vi "Main.vi"() -> ()   [LabVIEW 2014, in "CSV Analyzer.lvlib"]
uses:
  CSV Analyzer.lvlib
  <vilib>/SLL/SLL Table/SLL Table.lvclass
  <vilib>/Utility/error.llb/DialogType.ctl
  <vilib>/SLL/SLL Queued State Machine/Queue Driver/Create Queue.vi
  <vilib>/SLL/SLL Queued State Machine/Queue Driver/Enqueue an Item to Queue.vi
  <vilib>/SLL/SLL Queued State Machine/Queue Driver/Dequeue Queue.vi
  <vilib>/Utility/file.llb/Read From Spreadsheet File (string).vi
  <vilib>/SLL/SLL Queued State Machine/Queue Driver/Enqueue N Items.vi
  <vilib>/SLL/SLL Queued State Machine/Queue Driver/Flush Queue.vi
  <vilib>/SLL/SLL Queued State Machine/Queue Driver/Release Queue.vi
  <vilib>/SLL/SLL Queued State Machine/SLL QSM.lvlib
  <vilib>/SLL/SLL Spreadsheet/SLL Spreadsheet.lvlib
panel:
  in  "Delimiter":string(combo)=","
  in  "Use LabVIEW File Read?":bool
  in  "CSV File Path":path
  out "Total Columns":i32
  out "Total Rows":i32
  in  "Headers to List[]":string[](array[combo])
  in  "Filters":T1(array[cluster])
  out "Status":string
  in  "Count Rows":bool
  in  "Mini Table":bool
  out "Displayed Column Count":i32
  out "Displayed Row Count":i32
  in  "2D Data Out[][]":i32(listbox)
  # "CSV Analyzer"
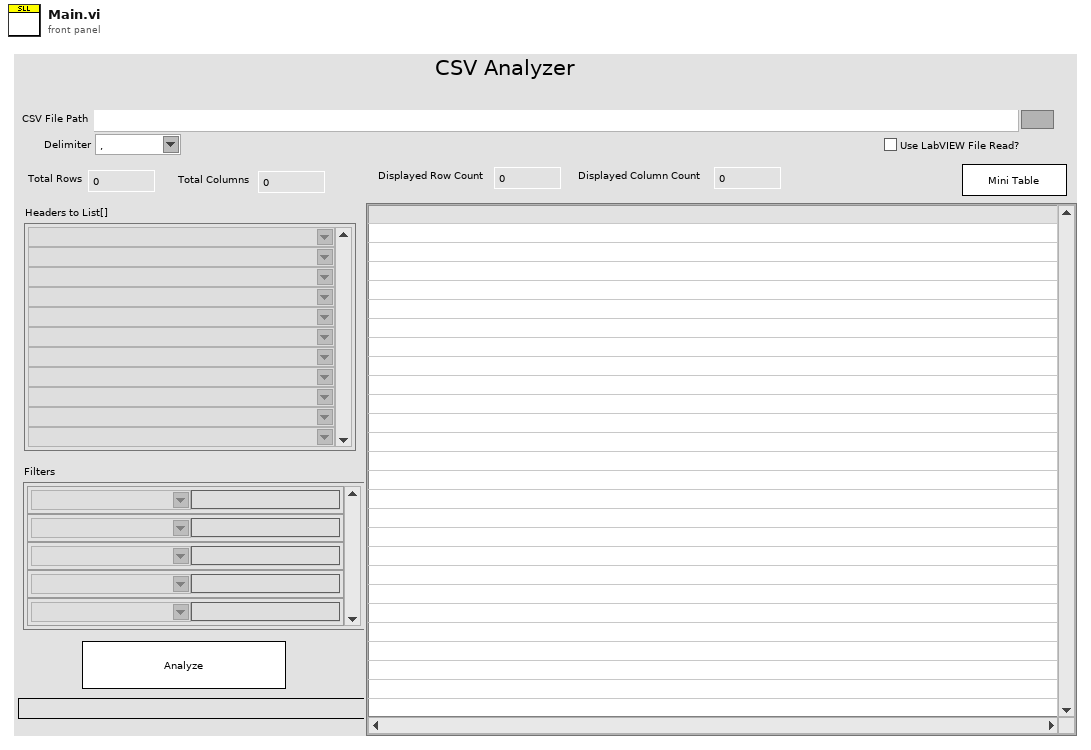
[diagram p1: front panel]
types:
  T1 = cluster{"Enable?":string, "Column Name":string}[]
  T2 = cluster{"Flags":cluster{"Source Code?":bool}, "SLL Table":refnum<class "SLL Table.lvclass">, "Headers[]":string[]}
  T3 = typedef "DialogType.ctl" = u16
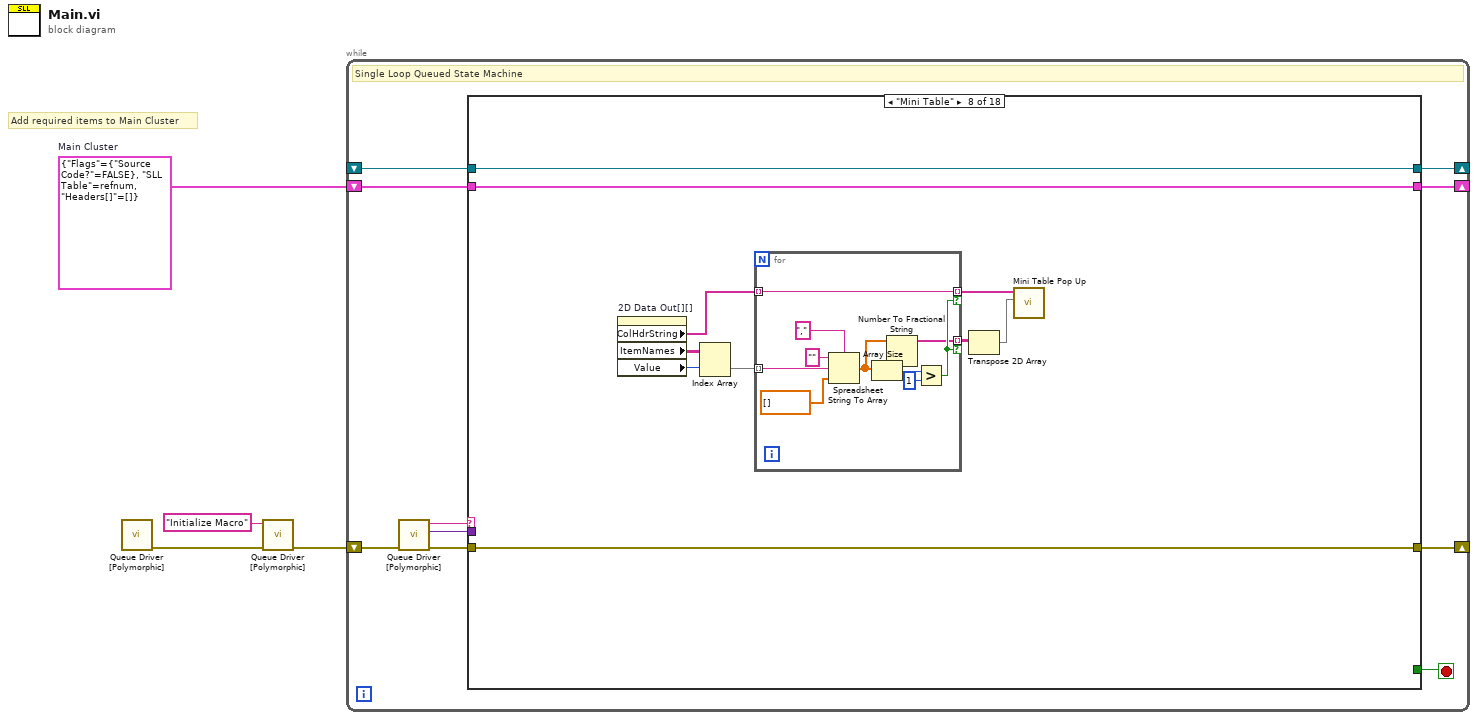
[diagram p0: block diagram]
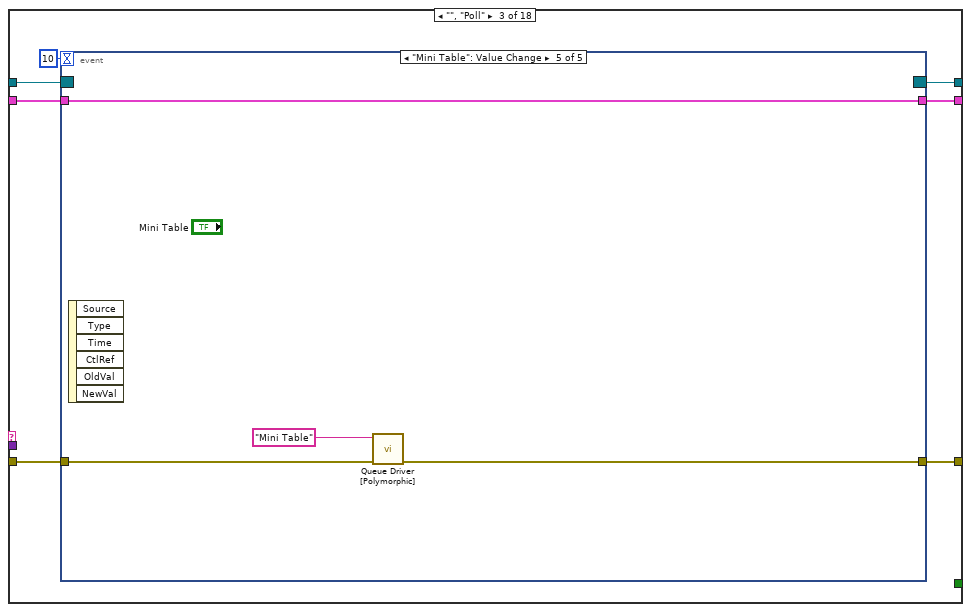
[diagram p4: hidden frame]
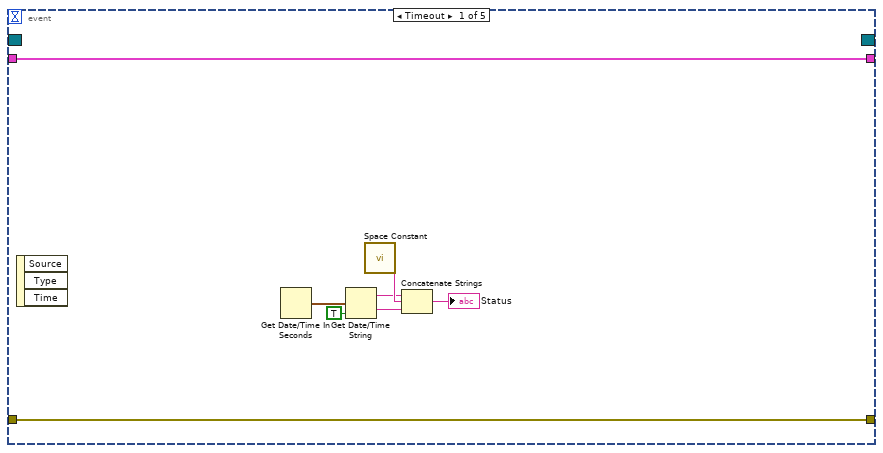
[diagram p5: hidden frame]
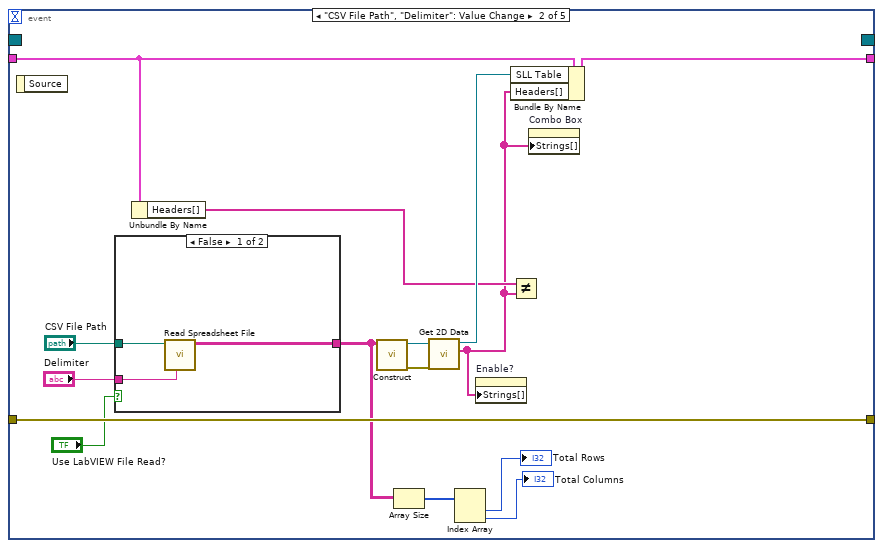
[diagram p6: hidden frame]
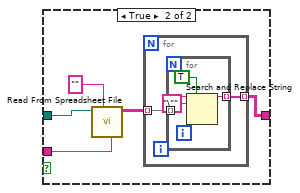
[diagram p7: hidden frame]
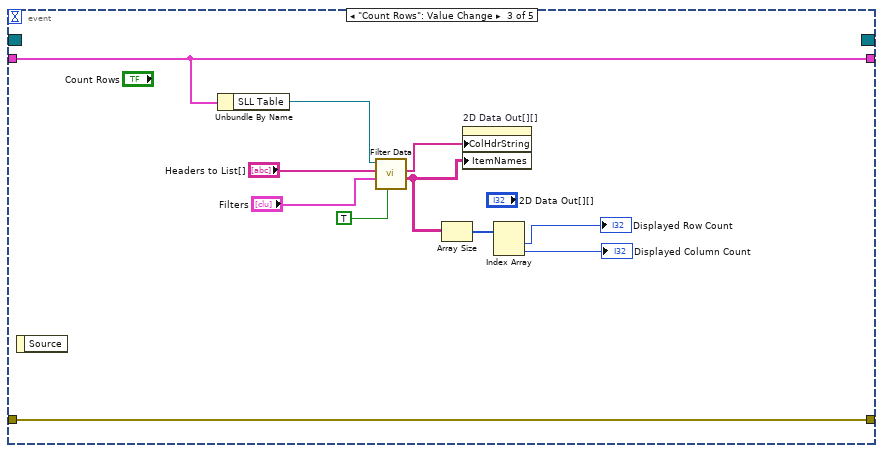
[diagram p8: hidden frame]
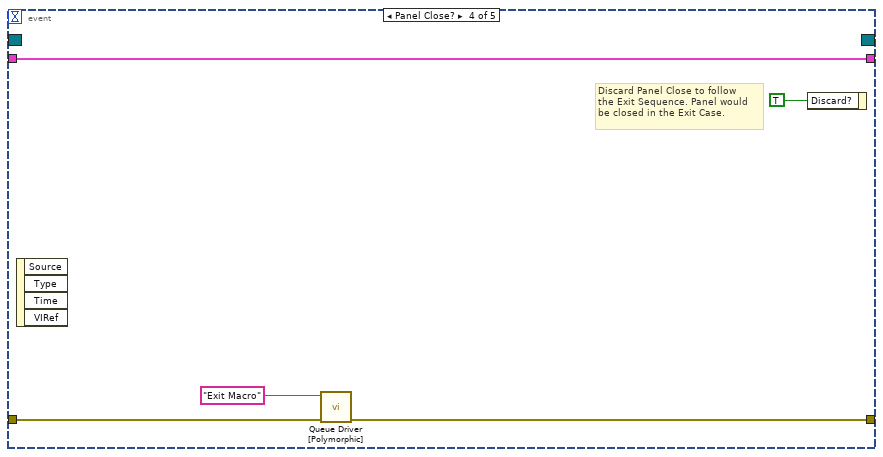
[diagram p9: hidden frame]
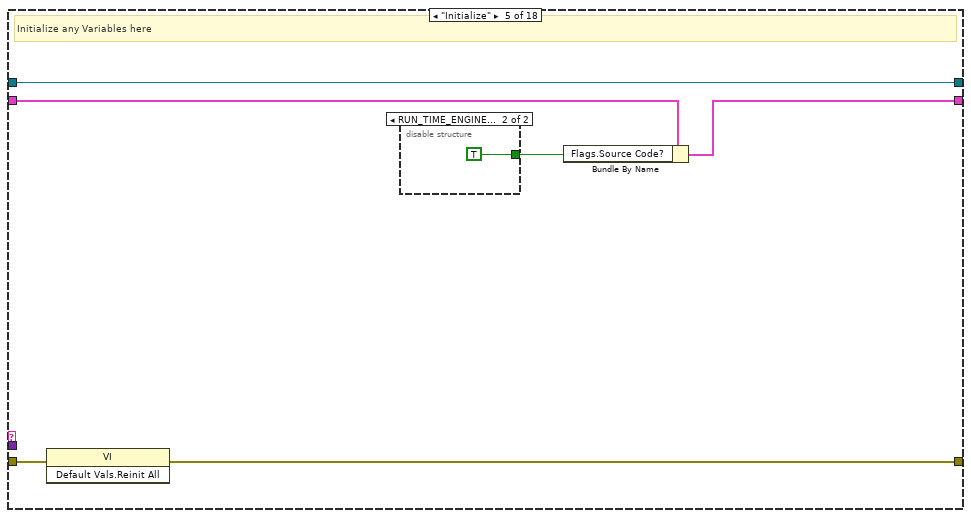
[diagram p11: hidden frame]
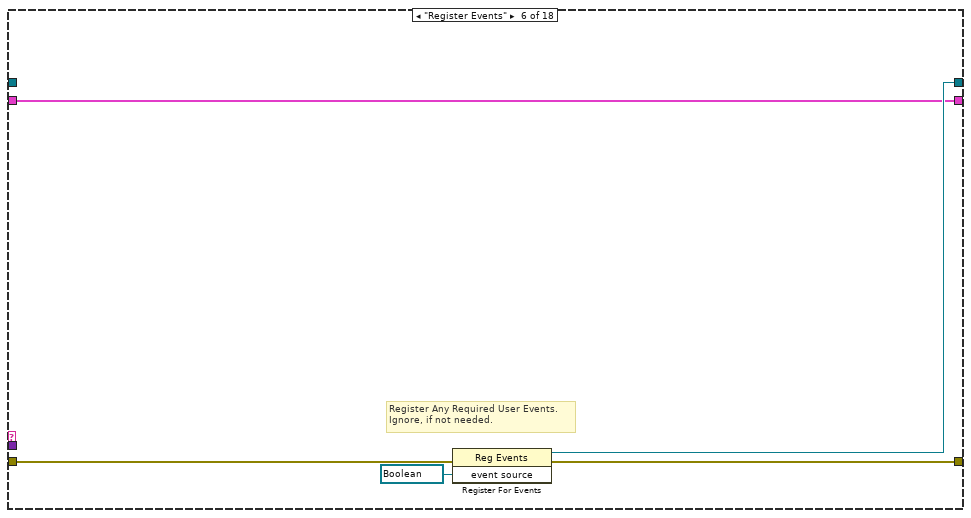
[diagram p13: hidden frame]
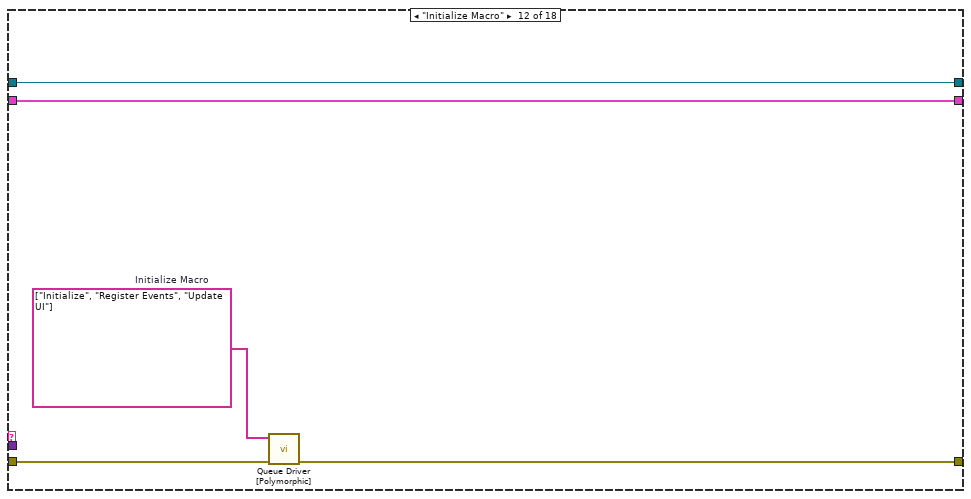
[diagram p18: hidden frame]
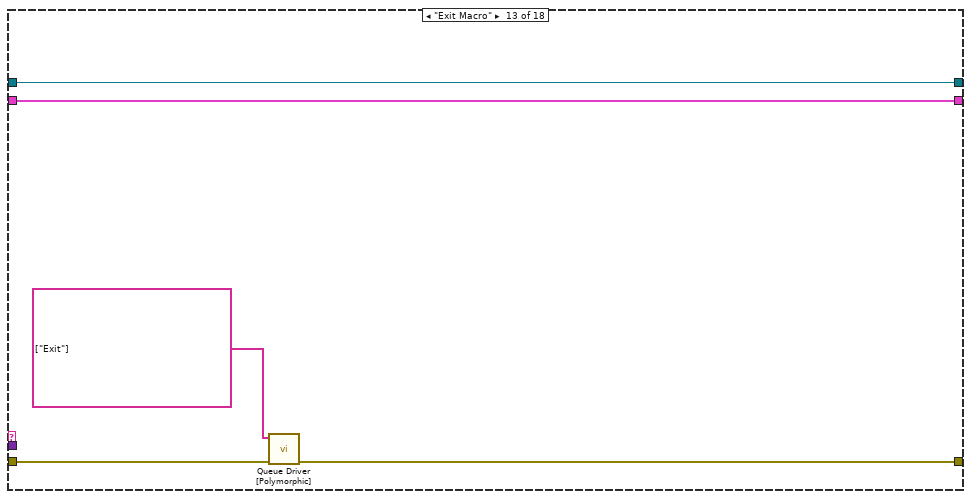
[diagram p19: hidden frame]
diagram:
  w3 = T2 {"Flags"={"Source Code?"=FALSE}, "SLL Table"=refnum, "Headers[]"=[]}  # Main Cluster
  # "Add required items to Main Cluster"
  n1 = call-poly <vilib>:"Queue Driver [Polymorphic].vi"() -> ("Error Out"=w2:errorcluster)  [unwired: 11 in]
  n2 = call-poly <vilib>:"Queue Driver [Polymorphic].vi"("Error In"=w2, "Item to Add"="Initialize Macro") -> ("Error Out"=w1:errorcluster)  [unwired: 9 in]
  n3 = while "SLL Queued State Machine" {
    shift-right: [w12] -> _
    shift-left: w1 -> [w14]
    shift-right: [w9] -> _
    shift-left: _ -> [w8]
    shift-right: [w7] -> _
    shift-left: w3 -> [w6]
    stop <- w11 stop-if-true
    # "Single Loop Queued State Machine"
    n4 = call-poly <vilib>:"Queue Driver [Polymorphic].vi"("Error In"=w14) -> ("Error Out"=w13:errorcluster, "Data"=w5:variant, "Dequeue"=w10:string)  [unwired: 8 in]
    n5 = case "QSM Case Structure" shown="\"Mini Table\"" w10 {
      selector: w10 -> [_ _ _ _ _ _ _ _ _ _ _ _ _ _ w148 _ _ _]
      tunnel: w13 -> [w17 w20 w25 w87 w88 w99 w102 w112 w125 w128 w131 w134 w139 w144 w147 w160 w163 w176]
      tunnel: [w17 w20 w26 w87 w89 w98 w102 w112 w125 w128 w131 w133 w138 w144 w151 w158 w163 w172] -> w12
      tunnel: [_ _ _ _ _ _ _ _ _ _ _ _ _ _ _ _ _ TRUE] -> w11
      tunnel: [w16 w19 w24 w86 w93 w97 w101 w111 w124 w127 w130 w136 w141 w143 w154 w157 w162 w175] -> w9
      tunnel: w8 -> [w16 w19 w23 w86 w93 _ w101 w111 w124 w127 w130 w136 w141 w143 w154 w157 w162 w175]
      tunnel: [w15 w18 w21 w85 w90 w96 w100 w110 w123 w126 w129 w135 w140 w142 w153 w156 w161 w174] -> w7
      tunnel: w6 -> [w15 w18 w22 w85 w91 w96 w100 w110 w123 w126 w129 w135 w140 w142 w153 w156 w161 w174]
      tunnel: w5 -> [_ _ _ _ _ _ _ _ _ _ _ _ _ _ _ _ _ _]
      frame "/--------------- Read Me -----------------/" {
        # "General Purpose Queue Based State Machine for Any Use Case (main application, module, pop up message etc)\n\nAdvantages:\n1. No Need to Pass Queue References between Queue Driver VIs.\n2. This template can be safely used in multiple parallel running modules without any issues.\n3. This template can also be safely used even in cases where the VI is configured to be a Clone, where multiple \ninstances of the VI could be executing concurrently.\n\nHow to Use:\n1. Add necessary items to the Main Cluster.\n2. Use the Polymorphic Queue Driver for doing any queue operations. There is no need to pass the queue driver\nreference, as the Queue Driver automatically infers the reference based on the VI instance from which it is called.\n3. Add any required user events in the \"Register Events\" case. Ignore if not needed.\n4. Use \"Sequences\" section for defining any list of state calls, which could be used in multiple places. \nEg: Initialize Sequence, might be needed if we need to any reinitialization."
      }
      frame "/------------------ Poll -------------------/" {
      }
      frame "", "Poll" {
        n6 = event shown="[4] \"Mini Table\": Value Change" {
          selector: w23 -> [_ _ _ _ _]
          dyn-events: [_ _ _ _ _] -> w24
          timeout: 10 -> [_ _ _ _ _]
          tunnel: [w35 w50 w75 w79 w83] -> w26
          tunnel: w25 -> [w35 w50 w75 w80 w84]
          tunnel: w22 -> [w34 w45 w74 w78 w82]
          tunnel: [w34 w47 w74 w78 w82] -> w21
          event Timeout {
            n7 = event-data() -> ()  [unwired: 1 in, 3 out]
            n8 = Get Date/Time In Seconds() -> (seconds since 1Jan1904=w33:timestamp)
            n9 = Get Date/Time String(seconds (now)=w33, want seconds? (F)=TRUE) -> (date string=w29:string, time string=w28:string)  [unwired: 1 in]
            n10 = call <vilib>:"Space Constant.vi"() -> ("String"=w30:string)
            n11 = Concatenate Strings(w29, w30, w28) -> (→"Status":string)
          }
          event "CSV File Path", "Delimiter": Value Change {
            n12 = event-data() -> ()  [unwired: 1 in, 1 out]
            n13 = case shown="False" "Use LabVIEW File Read?" {
              tunnel: [w53 w55] -> w42
              tunnel: "CSV File Path" -> [w52 w58]
              tunnel: "Delimiter" -> [w51 w54]
              frame False {
                n14 = call <vilib>:"Read Spreadsheet File.vi"("Delimiter (tab)"=w51, "File Path"=w52) -> ("2D Array"=w53:string[][])  [unwired: 8 in, 1 out]
              }
              frame True {
                n15 = call-poly <vilib>:"Read From Spreadsheet File.vi"("delimiter (\\t)"=w54, "format (%s)"="", "file path (dialog if empty)"=w58) -> ("all rows"=w56:string[][])  [unwired: 4 in, 4 out]
                n16 = for {
                  tunnel: w56 -> [w60] mode=indexing
                  tunnel: [w59] -> w55 mode=indexing
                  n17 = for {
                    tunnel: w60 -> [w64] mode=indexing
                    tunnel: [w62] -> w59 mode=indexing
                    n18 = Search and Replace String(replace all?=TRUE ("replace all? (F)"), input string=w64, search string="\"") -> (result string=w62:string)  [unwired: 5 in, 3 out]
                  }
                }
              }
            }
            n19 = Unbundle By Name(w45) -> ("Headers[]"=w44:string[])
            n20 = call <vilib>:"Construct.vi"("2D String with Headers"=w42) -> ("error out"=w49:errorcluster, "SLL Spreadsheet"=w48:refnum<class "SLL Table.lvclass">)  [unwired: 9 in]
            n21 = Array Size(array=w42) -> (size(s)=w41:i32[])
            n22 = call <vilib>:"Get 2D Data.vi"("error in (no error)"=w49, "SLL Spreadsheet in"=w48) -> ("Headers Out[]"=w38:string[], "SLL Spreadsheet out"=w46:refnum<class "SLL Table.lvclass">)  [unwired: 6 in, 2 out]
            n23 = Index Array(array=w41) -> (element #1=→"Total Rows":i32, element #2=→"Total Columns":i32)  [unwired: 2 in]
            n24 = property on="Enable?" class="CmbBox"("Strings[]"=w38) -> ()  [unwired: 2 in, 2 out]
            n25 = Bundle By Name(cluster=w45, "SLL Table"=w46, "Headers[]"=w38) -> (w47:T2)
            n26 = Not Equal?(x=w44, y=w38) -> ()  [unwired: 1 out]
            n27 = property on="Combo Box" class="CmbBox"("Strings[]"=w38) -> ()  [unwired: 2 in, 2 out]
          }
          event "Count Rows": Value Change {
            n28 = event-data() -> ()  [unwired: 1 in, 1 out]
            n29 = Unbundle By Name(w74) -> ("SLL Table"=w73:refnum<class "SLL Table.lvclass">)
            n30 = call <vilib>:"Filter Data.vi"("Count? (F)"=TRUE, "Value Filters[]"="Filters", "Header Order[]"="Headers to List[]", "SLL Table in"=w73) -> ("2D Data Out[][]"=w65:string[][], "Headers Out[]"=w71:string[])  [unwired: 4 in, 2 out]
            n31 = Array Size(array=w65) -> (size(s)=w70:i32[])
            n32 = property on="2D Data Out[][]" class="MCListbox (strict)"("ColHdrString"=w71, "ItemNames"=w65) -> ()  [unwired: 2 in, 2 out]
            n33 = Index Array(array=w70) -> (element #1=→"Displayed Row Count":i32, element #2=→"Displayed Column Count":i32)  [unwired: 2 in]
          }
          event Panel Close? {
            # "Discard Panel Close to follow\nthe Exit Sequence. Panel would\nbe closed in the Exit Case."
            n34 = event-data() -> ()  [unwired: 1 in, 4 out]
            n35 = call-poly <vilib>:"Queue Driver [Polymorphic].vi"("Error In"=w80, "Item to Add"="Exit Macro" ("Enqueue")) -> ("Error Out"=w79:errorcluster)  [unwired: 9 in]
            n36 = event-data("Discard?"=TRUE) -> ()  [unwired: 1 in, 1 out]
          }
          event "Mini Table": Value Change {
            n37 = event-data() -> ()  [unwired: 1 in, 6 out]
            n38 = call-poly <vilib>:"Queue Driver [Polymorphic].vi"("Error In"=w84, "Item to Add"="Mini Table" ("Enqueue")) -> ("Error Out"=w83:errorcluster)  [unwired: 9 in]
          }
        }
      }
      frame "/--------------- Initialize -----------------/" {
      }
      frame "Initialize" {
        # "Initialize any Variables here"
        n39 = invoke class="VI" method="Default Vals.Reinit All"(error in=w88) -> (error out=w89:errorcluster)  [unwired: 2 in, 2 out]
        n40 = disable-structure shown="RUN_TIME_ENGINE==False" {
          disable-tunnel: [_ TRUE] -> w92
          frame condition #0 {
          }
          frame condition #1 (active) {
          }
        }
        n41 = Bundle By Name(cluster=w91, "Flags.Source Code?"=w92) -> (w90:T2)
      }
      frame "Register Events" {
        # "Register Any Required User Events. \nIgnore, if not needed."
        n42 = register-events(error in=w99, refnum<vi> refnum ("event source")) -> (reference out=w97:refnum<event-registration>, error out=w98:errorcluster)  [unwired: 1 in]
      }
      frame "/---------- Custom Case Splitter ----------/" {
      }
      frame "Mini Table" {
        n43 = property on="2D Data Out[][]" class="MCListbox (strict)"() -> ("ColHdrString"=w106:string[], "ItemNames"=w109:string[][], "Value"=w108:i32)  [unwired: 2 in, 2 out]
        n44 = Index Array(array=w109, index (row)=w108) -> (element=w107:string[])  [unwired: 1 in]
        n45 = for {
          tunnel: w107 -> [w122] mode=indexing
          tunnel: w106 -> [w116] mode=indexing
          tunnel: [w113] -> w104 mode=indexing if=w115
          tunnel: [w116] -> w105 mode=indexing if=w115
          n46 = Spreadsheet String To Array(delimiter (Tab)=",", format string="", spreadsheet string=w122, array type (2D Dbl)=dbl[] []) -> (array=w117:dbl[])
          n47 = Array Size(array=w117) -> (size(s)=w119:i32)
          n48 = Number To Fractional String(number=w117) -> (F-format string=w113:string[])  [unwired: 3 in]
          n49 = Greater?(x=w119, y=1) -> (0:w115:bool)
        }
        n50 = Transpose 2D Array(2D array=w104) -> (transposed array=w103:string[][])
        n51 = call "Mini Table Pop Up.vi"("Data[][]"=w103, "Headers[]"=w105) -> ()  [unwired: 9 in, 1 out]
      }
      frame "/-------------- User Interface --------------/" {
        # "Duplicate this case to create additional case splitters for readability"
      }
      frame "Update UI" {
        # "Update Front Panel Controls in this Case"
      }
      frame "/----------------- Macros -----------------/" {
      }
      frame "Initialize Macro" {
        w132 = string[] ["Initialize", "Register Events", "Update UI"]  # Initialize Macro
        n52 = call-poly <vilib>:"Queue Driver [Polymorphic].vi"("Error In"=w134, "Enqueue N"=w132) -> ("Error Out"=w133:errorcluster)  [unwired: 9 in]
      }
      frame "Exit Macro" {
        n53 = call-poly <vilib>:"Queue Driver [Polymorphic].vi"("Error In"=w139, "Enqueue N"=string[] ["Exit"]) -> ("Error Out"=w138:errorcluster)  [unwired: 9 in]
      }
      frame "/-------------- Error Handler--------------/" {
      }
      frame Default {
        # "Undefined Case/Spelling Errors - Show Message to Developer"
        n54 = property class="VI"(error in=w147) -> (error out=w146:errorcluster, "Name"=w145:string)  [unwired: 1 in, 1 out]
        n55 = Format Into String(format string="\"%s\" in the VI - %s" ("message"), initial string="Undefined case - ", error in=w146, w148, w145) -> (resulting string=w149:string, error out=w151:errorcluster)
        n56 = One Button Dialog(message=w149) -> ()  [unwired: 1 in, 1 out]
      }
      frame "Error" {
        w155 = T3 2 items=["no dialog", "OK message", "continue or stop message", "OK message + warnings", "continue/stop + warnings"] ("type of dialog (OK msg:1)")
        # "Handle the Error"
        n57 = call <vilib>:"Simple Error Handler.vi"("type of dialog (OK msg:1)"=w155, "error in (no error)"=w160) -> ("error out"=w159:errorcluster)  [unwired: 3 in, 4 out]
        n58 = call <vilib>:"Clear Errors.vi"("error in (no error)"=w159) -> ("error out"=w158:errorcluster)  [unwired: 5 in, 1 out]
      }
      frame "/------------------- Exit --------------------/" {
      }
      frame "Exit" {
        n59 = call-poly <vilib>:"Queue Driver [Polymorphic].vi"("Error In"=w176) -> ("Error Out"=w177:errorcluster)  [unwired: 9 in, 1 out]
        n60 = Unbundle By Name(w174) -> ("Flags.Source Code?"=w167:bool)
        n61 = call-poly <vilib>:"Queue Driver [Polymorphic].vi"("Error In"=w177) -> ("Error Out"=w173:errorcluster)  [unwired: 10 in]
        n62 = Call Chain() -> (call chain=w171:string[])
        n63 = Array Size(array=w171) -> (size(s)=w170:i32)
        n64 = Equal?(x=w170, y=1) -> (x = y?=w168:bool)
        n65 = And(x=w167, y=w168) -> (x .and. y?=w166:bool)
        n66 = case "Skip Panel Close when in Source\nCode and is the top most caller" shown="True" w166 {
          tunnel: w173 -> [w180 w182]
          tunnel: [w181 w182] -> w172
          frame False {
            # "Close Panel"
            n67 = invoke class="VI" method="FP.Close"() -> (error out=w179:errorcluster)  [unwired: 3 in, 2 out]
            n68 = Merge Errors(w180, w179) -> (w181:errorcluster)
          }
          frame True {
            # "Do Not Close Panel"
          }
        }
        n69 = property on="2D Data Out[][]" class="MCListbox (strict)"("ColHdrString"=string[] [] ("Column Header Strings[]"), "ItemNames"=string[][] [] ("2D Data Out[][] 2")) -> ()  [unwired: 2 in, 2 out]
      }
    }
  }
